vi "Initialize-motors.vi"(8 "error in (no error)":errorcluster, 11 "Object ref in":T1) -> (0 "error out":errorcluster, 3 "Object ref out":T1)   [LabVIEW 2013, in "PowderDeposition.lvlib" / "PD-Main.lvclass"]
uses:
  PD-Main.lvclass
  Object-reference.ctl
  PD-Main.lvclass/PD-Main.ctl
  Assembly/Motor-assembly.lvclass
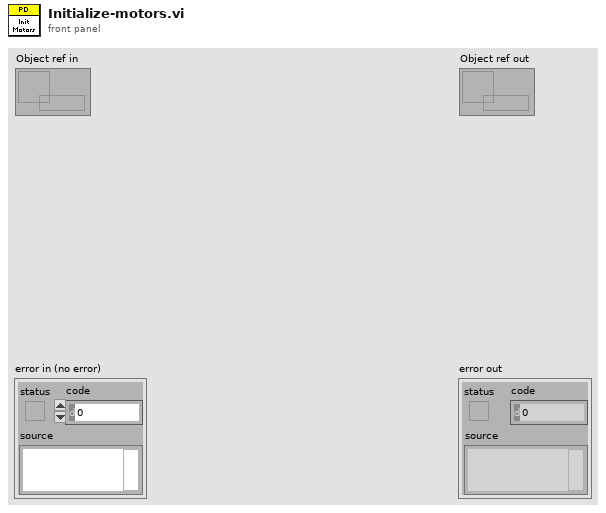
[diagram p1: front panel]
types:
  T1 = typedef "PowderDeposition.lvlib/PD-Main.lvclass/Object-reference.ctl" = refnum<data-value>
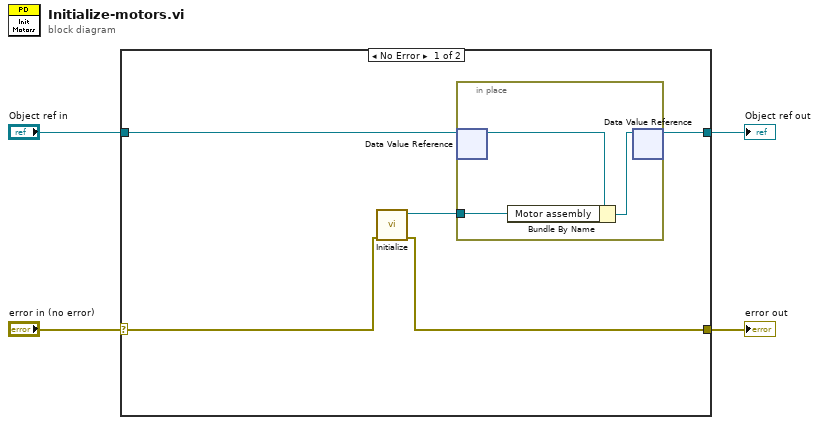
[diagram p0: block diagram]
diagram:
  n1 = case shown="No Error" "error in (no error)" {
    selector: "error in (no error)" -> [w9 w14]
    tunnel: [w8 w14] -> w3
    tunnel: [w6 w13] -> w1
    tunnel: "Object ref in" -> [w7 w13]
    frame No Error {
      n2 = call "Initialize.vi"("error in (no error)"=w9) -> ("error out"=w8:errorcluster, "Available motors out"=w5:refnum<class "Motor-assembly.lvclass">)  [unwired: 9 in]
      n3 = in-place {
        in-place-border: w5 -> [w10]
        n4 = in-place-dvr #1(w7) -> (w12:refnum<class "PD-Main.lvclass">)  [unwired: 1 out]
        n5 = Bundle By Name(cluster=w12, "Motor assembly"=w10) -> (w11:refnum<class "PD-Main.lvclass">)
        n6 = in-place-dvr #1(w11) -> (w6:T1)  [unwired: 1 out]
      }
    }
    frame Error {
    }
  }
  "error out" <- w3
  "Object ref out" <- w1
